vi "configure.vi"(8 "error in (no error)":errorcluster, 11 "StimulatorDL090824Gate in":refnum<class "StimulatorDL090824Gate.lvclass">) -> (0 "error out":errorcluster, 3 "StimulatorDL090824Gate out":refnum<class "StimulatorDL090824Gate.lvclass">)   [LabVIEW 2010, in "StimulatorDL090824Gate.lvclass"]
doc: "The dynamic dispatch version of this VI loads and displays the configuration file associated with the plug-in object. The user modify and save the configuration data."
uses:
  StimulatorDL090824Gate.lvclass
  common/xcontrols/XComponentSpecification/XComponentSpecification/XComponentSpecification.xctl
  StimulatorDL090824Gate.lvclass/StimulatorDL090824Gate.ctl
  Clock/GenericClock/GenericClock/GenericClock.lvclass
  common/classes/GenericComponent/GenericComponent/GenericComponent.lvclass
panel:
  in  "clock spec":T1(xcontrol)
  in  "save button":bool
  in  "cancel button":bool
  out "configuration":string
  # "Configure StimulatorDL090824Gate"
  # "timing clock"
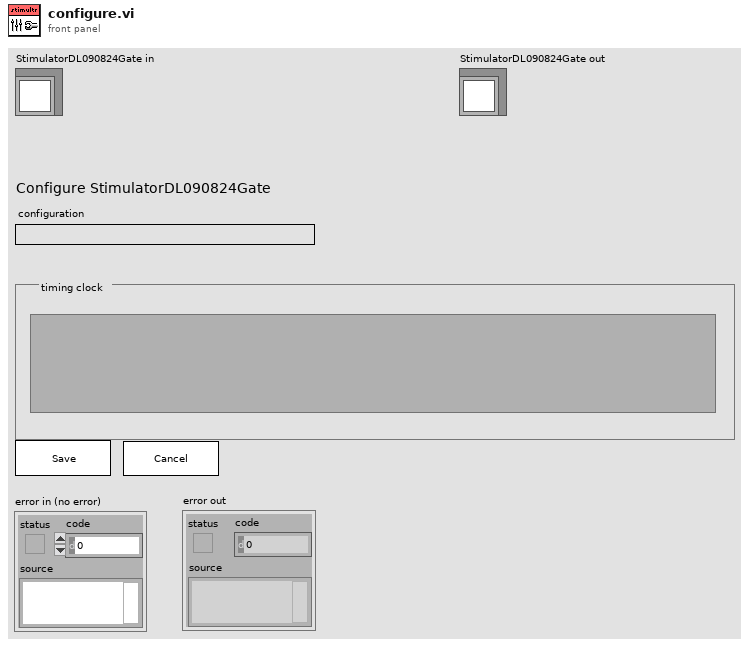
[diagram p1: front panel]
types:
  T1 = cluster{"class path":string, "configuration":string, "label":string, "settings name":string}
  T2 = typedef "plugin_specification.ctl" = cluster{"class path":string, "configuration":string, "label":string, "settings name":string}
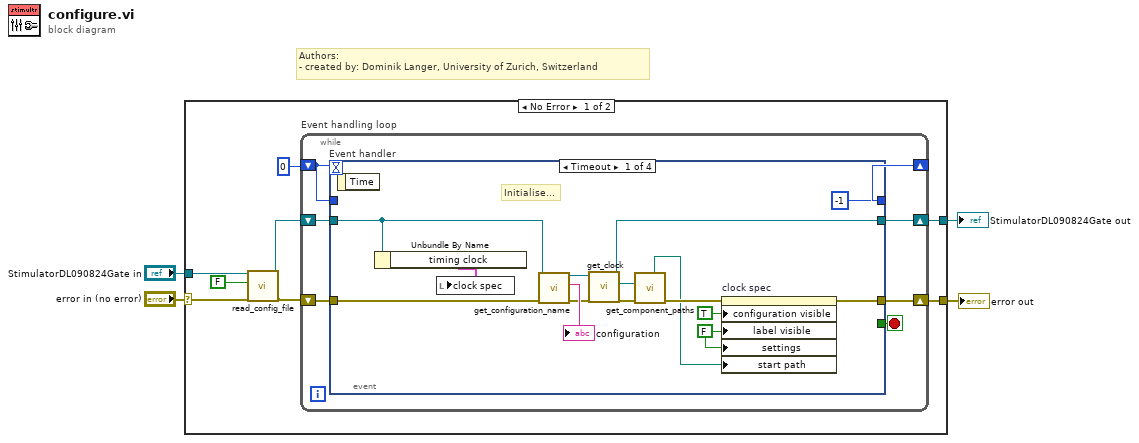
[diagram p0: block diagram]
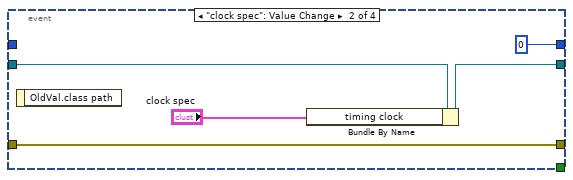
[diagram p2: hidden frame]
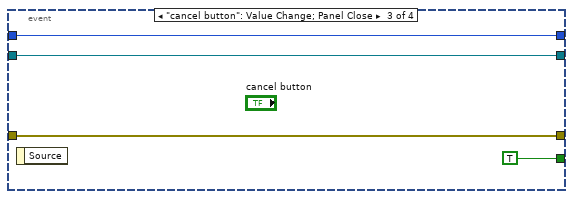
[diagram p3: hidden frame]
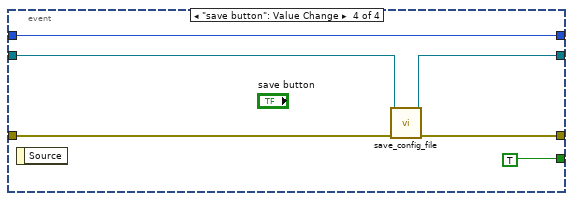
[diagram p4: hidden frame]
diagram:
  # "Authors: \n- created by: Dominik Langer, University of Zurich, Switzerland"
  n1 = case shown="No Error" "error in (no error)" {
    selector: "error in (no error)" -> [w8 w51]
    tunnel: [w12 w51] -> w2
    tunnel: "StimulatorDL090824Gate in" -> [w6 w50]
    tunnel: [w10 w50] -> w1
    frame No Error {
      n2 = call-dynamic "read_config_file.vi"("error in (no error)"=w8, "force load?"=FALSE, "GenericPlugin in"=w6) -> ("error out"=w7:errorcluster, "GenericPlugin out"=w5:refnum<class "StimulatorDL090824Gate.lvclass">)  [unwired: 7 in]
      n3 = while "Event handling loop" {
        shift-right: [w18] -> w12
        shift-left: w7 -> [w19]
        shift-right: [w16] -> _
        shift-left: 0 -> [w17]
        shift-right: [w13] -> w10
        shift-left: w5 -> [w14]
        stop <- w15 stop-if-true
        n4 = event "Event handler" shown="[0] Timeout" {
          selector: _ -> [_ _ _ _]
          dyn-events: _ -> [_ _ _ _]
          timeout: w17 -> [_ _ _ _]
          tunnel: w19 -> [w25 w36 w43 w47]
          tunnel: [w23 w36 w43 w45] -> w18
          tunnel: w17 -> [_ _ w42 w49]
          tunnel: [-1 0 w42 w49] -> w16
          tunnel: [_ _ TRUE TRUE] -> w15
          tunnel: w14 -> [w33 w39 w40 w44]
          tunnel: [w29 w38 w40 w46] -> w13
          event Timeout {
            w20 = FALSE ("configuration visible")
            # "Initialise..."
            n5 = event-data() -> ()  [unwired: 2 out]
            n6 = Unbundle By Name(w33) -> ("timing clock"=w26:T2)
            n7 = local write "clock spec"(w26) -> ()
            n8 = call "get_configuration_name.vi"("error in (no error)"=w25, "GenericPlugin.lvclass in"=w33) -> ("error out"=w31:errorcluster, "configuration name"=→"configuration":string, "GenericPlugin.lvclass out"=w30:refnum<class "StimulatorDL090824Gate.lvclass">)  [unwired: 7 in]
            n9 = call-dynamic "get_clock.vi"("error in (no error)"=w31, "Stimulator090724Scaffold in"=w30) -> ("error out"=w27:errorcluster, "clock"=w28:refnum<class "GenericClock.lvclass">, "Stimulator090724Scaffold out"=w29:refnum<class "StimulatorDL090824Gate.lvclass">)  [unwired: 7 in]
            n10 = call-dynamic "get_component_paths.vi"("error in (no error)"=w27, "GenericComponent in"=w28) -> ("error out"=w24:errorcluster, "component type directory"=w22:path)  [unwired: 4 in, 4 out]
            n11 = property on="clock spec" class="XComponentSpecification (strict"(error in=w24, "configuration visible"=TRUE, "label visible"=w20, "settings"=w20, "start path"=w22) -> (error out=w23:errorcluster)  [unwired: 1 in, 1 out]
          }
          event "clock spec": Value Change {
            n12 = event-data() -> ()  [unwired: 2 out]
            n13 = Bundle By Name(cluster=w39, "timing clock"="clock spec") -> (w38:refnum<class "StimulatorDL090824Gate.lvclass">)
          }
          event "cancel button": Value Change; Panel Close {
            n14 = event-data() -> ()  [unwired: 2 out]
          }
          event "save button": Value Change {
            n15 = event-data() -> ()  [unwired: 2 out]
            n16 = call-dynamic "save_config_file.vi"("error in (no error)"=w47, "GenericPlugin in"=w44) -> ("error out"=w45:errorcluster, "GenericPlugin out"=w46:refnum<class "StimulatorDL090824Gate.lvclass">)  [unwired: 8 in]
          }
        }
      }
    }
    frame Error {
    }
  }
  "error out" <- w2
  "StimulatorDL090824Gate out" <- w1
